vi "Draw XY Graph.vi"(5 "Plot Path":bool=TRUE, 7 "Plot Obstacles":bool=TRUE, 8 "error in (no error)":errorcluster, 10 "LIDAR Scan":u32[](array[numeric]), 11 "Simulator in":refnum<class "Simulator.lvclass">) -> (0 "error out":errorcluster, 2 "XY Graph":cluster{dbl[], dbl[]}[](graph), 3 "Simulator out":refnum<class "Simulator.lvclass">)   [LabVIEW 2011, in "Simulator.lvclass"]
uses:
  Simulator.lvclass
  LIDAR Scan To Plot.llb/LIDAR Characteristics.ctl
  Simulator.lvclass/Simulator.ctl
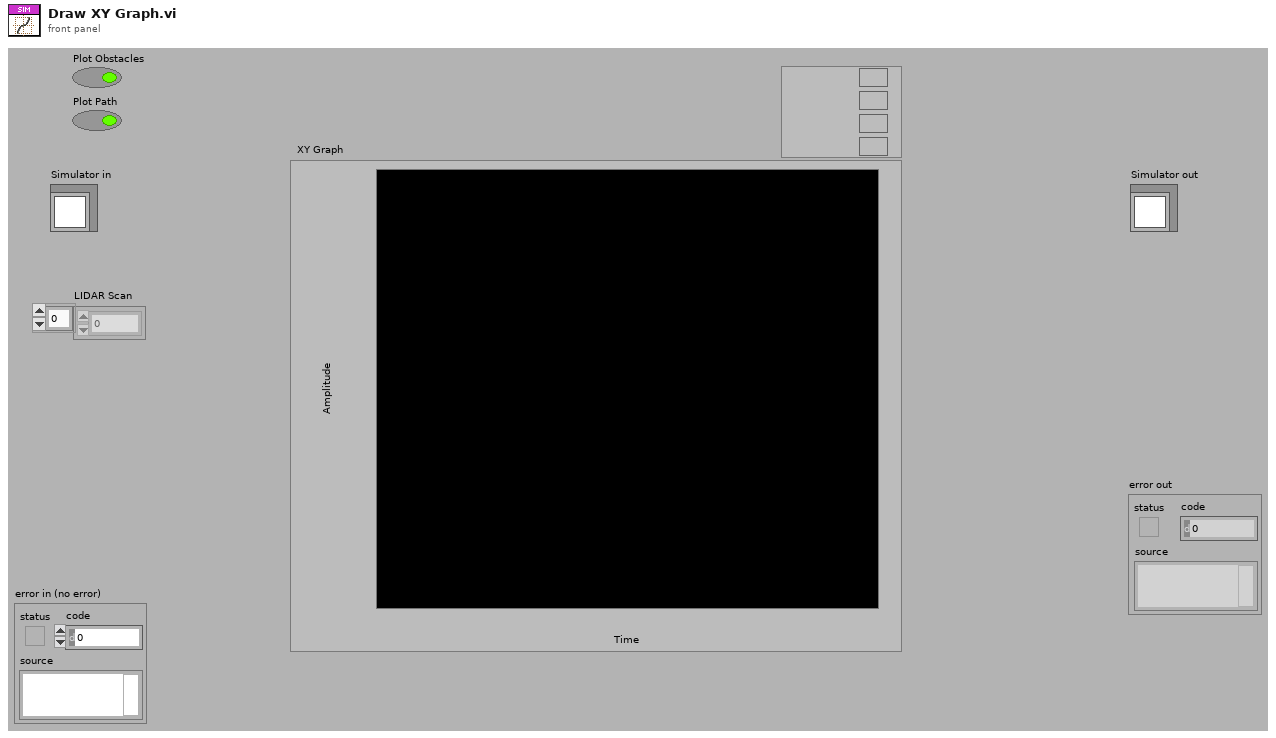
[diagram p1: front panel]
types:
  T1 = cluster{"Position Diff":dbl[], "Angle Diff (Rad)":dbl}
  T2 = typedef "LIDAR Characteristics.ctl" = cluster{"# of Sectors":i32, "Field of View":i32}
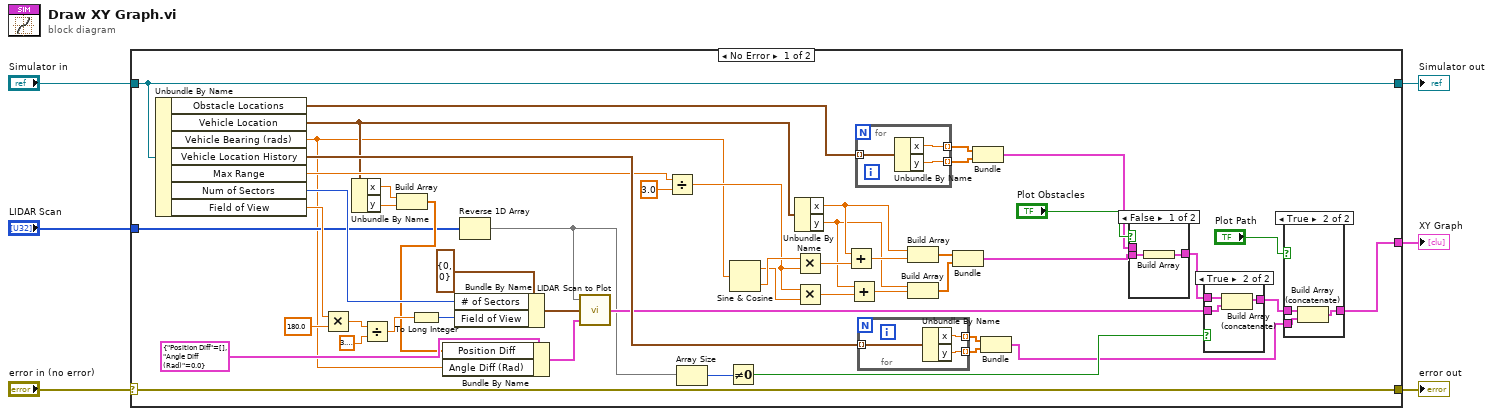
[diagram p0: block diagram]
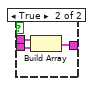
[diagram p3: hidden frame]
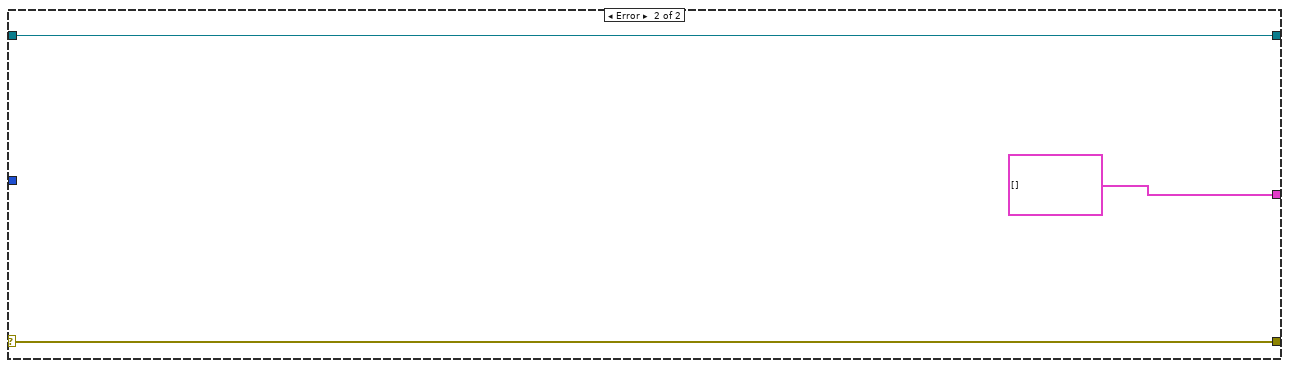
[diagram p5: hidden frame]
diagram:
  n1 = case shown="No Error" "error in (no error)" {
    selector: "error in (no error)" -> [w56 w78]
    tunnel: [w56 w78] -> w5
    tunnel: [w55 w77] -> w3
    tunnel: "Simulator in" -> [w55 w77]
    tunnel: [w9 cluster{dbl[], dbl[]}[] []] -> w2
    tunnel: "LIDAR Scan" -> [w19 _]
    frame No Error {
      n2 = Unbundle By Name(w55) -> ("Obstacle Locations"=w54:cluster{"x":dbl, "y":dbl}[], "Vehicle Location"=w23:cluster{"x":dbl, "y":dbl}, "Vehicle Bearing (rads)"=w16:dbl, "Vehicle Location History"=w47:cluster{"x":dbl, "y":dbl}[], "Max Range"=w46:dbl, "Num of Sectors"=w32:i32, "Field of View"=w31:dbl)
      n3 = Multiply(x=w31, y=180.0) -> (x*y=w29:dbl)
      n4 = Unbundle By Name(w23) -> ("x"=w22:dbl, "y"=w21:dbl)
      n5 = Divide(x=w29, y=3.141592653589793) -> (x/y=w27:dbl)
      n6 = Build Array(w22, w21) -> (w20:dbl[])
      n7 = To Long Integer(number=w27) -> (32bit integer=w26:i32)
      n8 = Bundle By Name(cluster=T1 {"Position Diff"=[], "Angle Diff (Rad)"=0.0} ("Difference from Ref Frame"), "Position Diff"=w20, "Angle Diff (Rad)"=w16) -> (w24:T1)
      n9 = Bundle By Name(cluster=T2 {"# of Sectors"=0, "Field of View"=0} ("LIDAR Characteristics"), "# of Sectors"=w32, "Field of View"=w26) -> (w34:T2)
      n10 = Reverse 1D Array(array=w19) -> (reversed array=w15:u32[])
      n11 = call "LIDAR Scan to Plot.vi"("Difference from Ref Frame"=w24, "LIDAR Characteristics"=w34, "LIDAR Scan"=w15) -> ("Translated LIDAR Plot"=w35:cluster{dbl[], dbl[]})  [unwired: 1 in, 1 out]
      n12 = Divide(x=w46, y=3.0) -> (x/y=w44:dbl)
      n13 = Array Size(array=w15) -> (size(s)=w18:i32)
      n14 = Not Equal To 0?(x=w18) -> (x != 0?=w17:bool)
      n15 = Sine & Cosine(0:w16) -> (1:w37:dbl, 2:w49:dbl)
      n16 = Unbundle By Name(w23) -> ("x"=w41:dbl, "y"=w38:dbl)
      n17 = Multiply(x=w49, y=w44) -> (x*y=w48:dbl)
      n18 = Multiply(x=w44, y=w37) -> (x*y=w36:dbl)
      n19 = Add(x=w41, y=w48) -> (x+y=w40:dbl)
      n20 = Add(x=w38, y=w36) -> (x+y=w39:dbl)
      n21 = for {
        tunnel: w54 -> [w75] mode=indexing
        tunnel: [w74] -> w53 mode=indexing
        tunnel: [w73] -> w52 mode=indexing
        n22 = Unbundle By Name(w75) -> ("x"=w74:dbl, "y"=w73:dbl)
      }
      n23 = for {
        tunnel: w47 -> [w72] mode=indexing
        tunnel: [w71] -> w43 mode=indexing
        tunnel: [w70] -> w42 mode=indexing
        n24 = Unbundle By Name(w72) -> ("x"=w71:dbl, "y"=w70:dbl)
      }
      n25 = Build Array(w41, w40) -> (w51:dbl[])
      n26 = Build Array(w38, w39) -> (w50:dbl[])
      n27 = Bundle(w51, w50) -> (w7:cluster{dbl[], dbl[]})  [unwired: 1 in]
      n28 = Bundle(w53, w52) -> (w8:cluster{dbl[], dbl[]})  [unwired: 1 in]
      n29 = Bundle(w43, w42) -> (w10:cluster{dbl[], dbl[]})  [unwired: 1 in]
      n30 = case shown="False" "Plot Obstacles" {
        tunnel: w7 -> [w62 w64]
        tunnel: [w61 w65] -> w14
        tunnel: w8 -> [_ w63]
        frame False {
          n31 = Build Array(w62) -> (w61:cluster{dbl[], dbl[]}[])
        }
        frame True {
          n32 = Build Array(w63, w64) -> (w65:cluster{dbl[], dbl[]}[])
        }
      }
      n33 = case shown="True" w17 {
        tunnel: w14 -> [w66 w69]
        tunnel: [w66 w68] -> w11
        tunnel: w35 -> [_ w67]
        frame False {
        }
        frame True {
          n34 = Build Array (concatenate)(w69, w67) -> (w68:cluster{dbl[], dbl[]}[])
        }
      }
      n35 = case shown="True" "Plot Path" {
        tunnel: w11 -> [w57 w60]
        tunnel: [w57 w59] -> w9
        tunnel: w10 -> [_ w58]
        frame False {
        }
        frame True {
          n36 = Build Array (concatenate)(w60, w58) -> (w59:cluster{dbl[], dbl[]}[])
        }
      }
    }
    frame Error {
    }
  }
  "error out" <- w5
  "Simulator out" <- w3
  "XY Graph" <- w2
